vi "Scripting.vi"() -> ()   [LabVIEW 2020]
uses:
  <vilib>/Utility/error.llb/DialogType.ctl
  <userlib>/_OpenG.lib/appcontrol/appcontrol.llb/Close Generic Object Refnum (Array)__ogtk.vi
  <userlib>/_OpenG.lib/appcontrol/appcontrol.llb/openg_application_control.lvlib
panel:
  out "array":string[][](array[string])
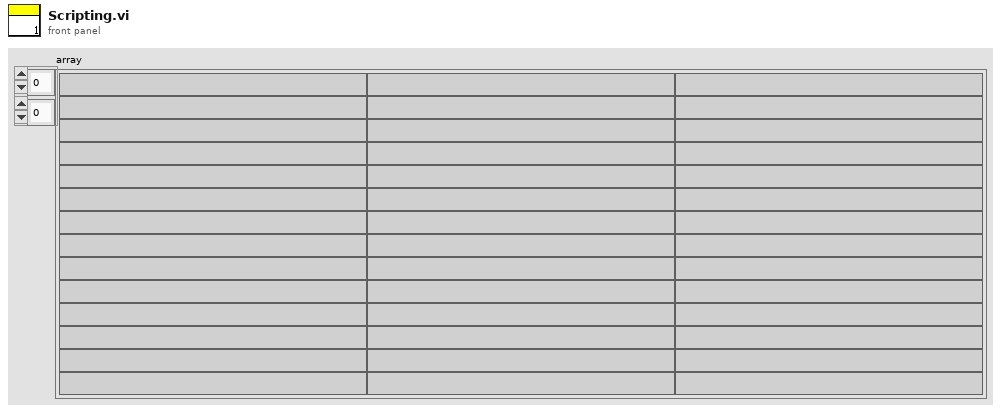
[diagram p1: front panel]
types:
  T1 = typedef "DialogType.ctl" = u16
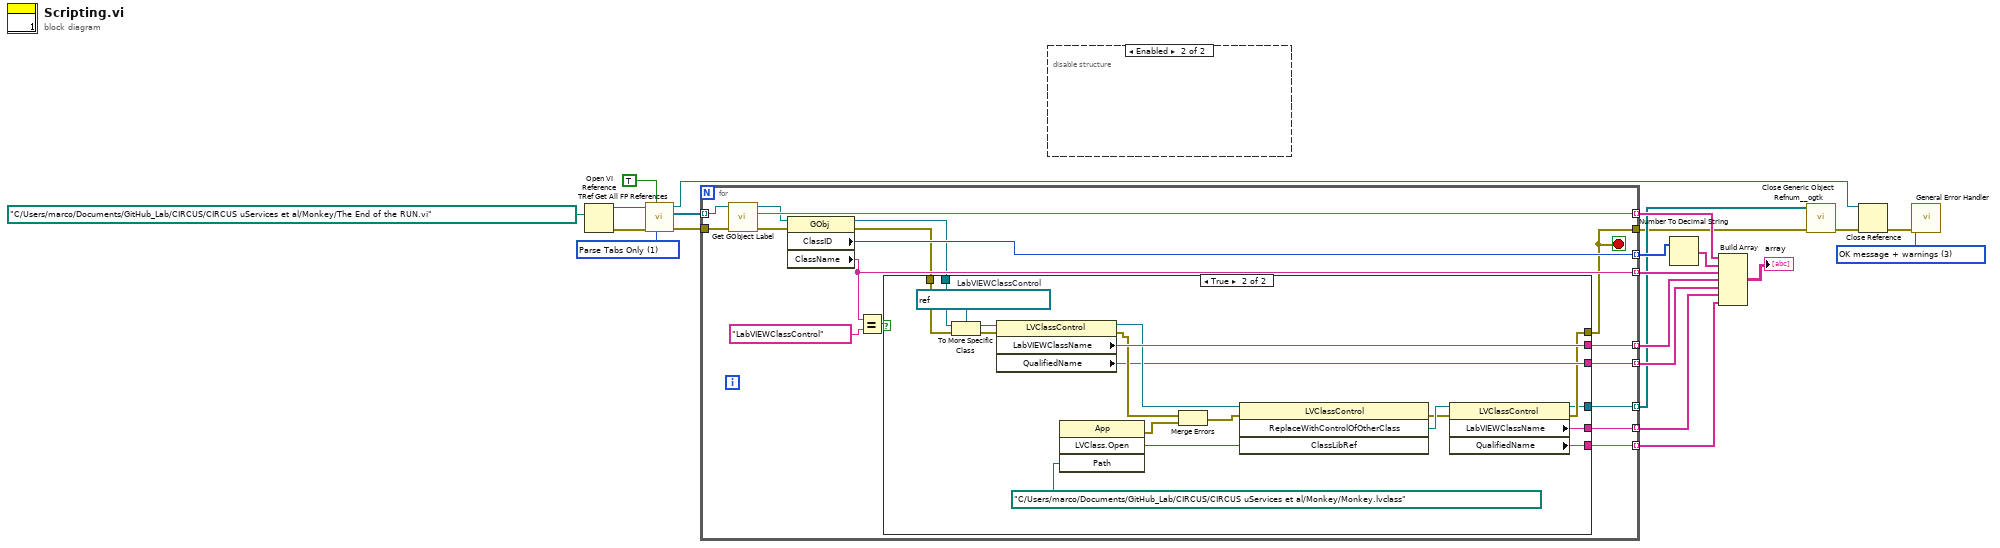
[diagram p0: block diagram]
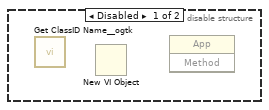
[diagram p2: hidden frame]
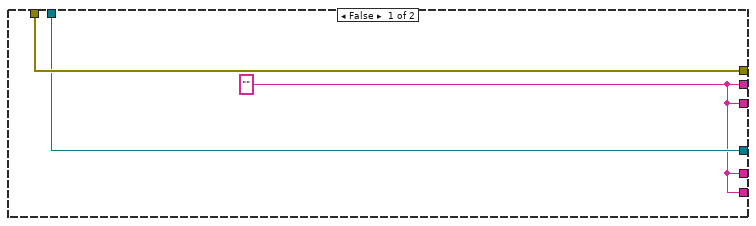
[diagram p3: hidden frame]
diagram:
  w13 = T1 3 items=["no dialog", "OK message", "continue or stop message", "OK message + warnings", "continue/stop + warnings"] ("type of dialog (OK msg:1)")
  w18 = u16 1 items=["Parse All", "Parse Tabs Only"] ("Parsing Rule")
  n1 = Open VI Reference(vi path=path "C:/Users/marco/Documents/GitHub_Lab/CIRCUS/CIRCUS uServices et al/Monkey/The End of the RUN.vi") -> (vi reference=w21:refnum<vi>, error out=w19:errorcluster)  [unwired: 5 in]
  n2 = call <vilib>:"TRef Get All FP References.vi"("Parsing Rule"=w18, "Ignore Decorations?"=TRUE, "error in (no error)"=w19, "VI Refnum"=w21) -> ("error out"=w15:errorcluster, "All FP Objects"=w16:refnum<vi>[], "dup VI Refnum"=w20:refnum<vi>)  [unwired: 3 in, 2 out]
  n3 = for {
    tunnel: w16 -> [w38] mode=indexing
    tunnel: w15 -> [w39]
    tunnel: [w37] -> w12 mode=indexing
    tunnel: [w28] -> w2
    tunnel: [w36] -> w10 mode=indexing
    tunnel: [w33] -> w11 mode=indexing
    tunnel: [w27] -> w7 mode=indexing
    tunnel: [w26] -> w6 mode=indexing
    tunnel: [w25] -> w5 mode=indexing
    tunnel: [w24] -> w4 mode=indexing
    tunnel: [w23] -> w3 mode=indexing
    stop <- w28 stop-if-true
    n4 = call <vilib>:"Get GObject Label.vi"("error in (no error)"=w39, "GObject"=w38) -> ("error out"=w34:errorcluster, "Object Label"=w37:string, "dup GObject"=w35:refnum<vi>)  [unwired: 5 in, 2 out]
    n5 = property class="GObj"(reference=w35, error in=w34) -> (reference out=w29:refnum<vi>, error out=w30:errorcluster, "ClassID"=w36:u32, "ClassName"=w33:string)
    n6 = Equal?(x=w33, y="LabVIEWClassControl") -> (x = y?=w31:bool)
    n7 = case shown="True" w31 {
      tunnel: w29 -> [w41 w61]
      tunnel: w30 -> [w42 w59]
      tunnel: [w40 w56] -> w27
      tunnel: [w40 w53] -> w26
      tunnel: [w42 w47] -> w28
      tunnel: [w40 w49] -> w25
      tunnel: [w40 w48] -> w24
      tunnel: [w41 w46] -> w23
      frame False {
        w40 = "" ("LabVIEWClassName")
      }
      frame True {
        w60 = refnum<vi> refnum  # LabVIEWClassControl
        n8 = To More Specific Class(target class=w60, reference=w61, error in=w59) -> (specific class reference=w58:refnum<vi>, error out=w57:errorcluster)
        n9 = property class="LVClassControl"(reference=w58, error in=w57) -> (reference out=w55:refnum<vi>, error out=w54:errorcluster, "LabVIEWClassName"=w56:string, "QualifiedName"=w53:string)
        n10 = invoke class="App" method="LVClass.Open"("Path"=path "C:/Users/marco/Documents/GitHub_Lab/CIRCUS/CIRCUS uServices et al/Monkey/Monkey.lvclass") -> (error out=w44:errorcluster, "LVClass.Open"=w45:refnum<vi>)  [unwired: 3 in, 2 out]
        n11 = Merge Errors(w54, w44) -> (w52:errorcluster)
        n12 = invoke class="LVClassControl" method="ReplaceWithControlOfOtherClass"(reference=w55, error in=w52, "ClassLibRef"=w45) -> (error out=w50:errorcluster, "ReplaceWithControlOfOtherClass"=w51:refnum<vi>)  [unwired: 1 in, 2 out]
        n13 = property class="LVClassControl"(reference=w51, error in=w50) -> (reference out=w46:refnum<vi>, error out=w47:errorcluster, "LabVIEWClassName"=w49:string, "QualifiedName"=w48:string)
      }
    }
  }
  n14 = disable-structure shown="Enabled" {
    frame Disabled {
      n15 = call <userlib>:"Get ClassID Name__ogtk.vi"() -> ()  [unwired: 8 in, 4 out]
      n16 = New VI Object() -> ()  [unwired: 8 in, 2 out]
      n17 = invoke class="App" method=#-1() -> ()  [unwired: 3 in, 3 out]
    }
    frame Enabled {
    }
  }
  n18 = Number To Decimal String(number=w10) -> (decimal integer string=w9:string[])  [unwired: 1 in]
  n19 = Build Array(w12, w9, w11, w7, w6, w5, w4) -> (→"array":string[][])
  n20 = call-poly <userlib>:"Close Generic Object Refnum__ogtk.vi"("error in (no error)"=w2, "Gen Refnum Array"=w3) -> ("error out"=w1:errorcluster)  [unwired: 9 in]
  n21 = Close Reference(reference=w20, error in (no error)=w1) -> (error out=w14:errorcluster)
  n22 = call <vilib>:"General Error Handler.vi"("type of dialog (OK msg:1)"=w13, "error in (no error)"=w14) -> ()  [unwired: 9 in, 5 out]
